vi "Stufentabelle umkehren.vi"(8 "error in (no error)":errorcluster caption="Fehler (Eingang, kein Fehler)") -> (0 "error out":errorcluster caption="Fehler (Ausgang)")   [LabVIEW 2020, in "Linearisierung v2.lvlib"]
uses:
  Linearisierung v2.lvlib
  Aktion Lin Daten aufarbeiten.ctl
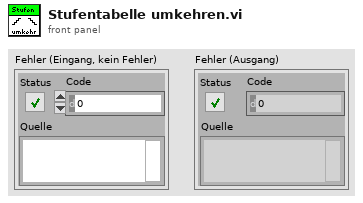
[diagram p1: front panel]
types:
  T1 = typedef "Linearisierung v2.lvlib/Aktion Lin Daten aufarbeiten.ctl" = enum16{"lesen", "Protkolldaten", "speichern", "laden", "EPA auswerten", "Tabelle schreiben", "Lin auswerten", "Tab init", "Stufentabelle", "EPA aktiviert", "Nachbehandlung laden", "Tabelle löschen", "Istwerte löschen", "Zeile löschen", "Zeile einfügen", "LIN aktiviert", "LIN/EPA aktiv laden", "EGAK Tab", "LIN übernehmen", "Tab init ohne Stufen"}
  T2 = typedef "Linearisierung v2.lvlib/Gasteiler.lvlib/Stufen Tabelle.ctl" = string[][]
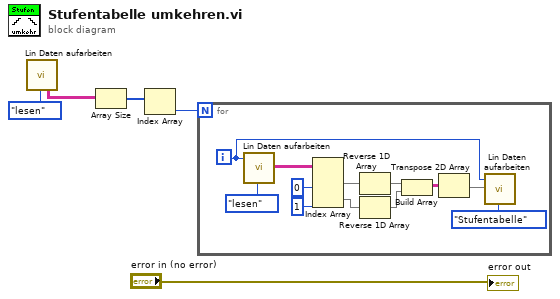
[diagram p0: block diagram]
diagram:
  n1 = call "Lin Daten aufarbeiten.vi"("Aktionen"=Aktion_Lin_Daten_aufarbeiten."lesen") -> ("TabellenArray"=w4:string[][][])  [unwired: 16 in, 10 out]
  n2 = Array Size(array=w4) -> (size(s)=w3:i32[])
  n3 = Index Array(array=w3) -> (element=w2:i32)  [unwired: 1 in]
  n4 = for {
    N: w2 -> [_]
    i -> [w15]
    n5 = call "Lin Daten aufarbeiten.vi"("Index (Seite)"=w15, "Aktionen"=Aktion_Lin_Daten_aufarbeiten."lesen") -> ("Stufen Tabelle"=w14:T2)  [unwired: 15 in, 10 out]
    n6 = Index Array(array=w14, index (col) #1=0 ("Deaktivierter Index (Spalte)"), index (col) #2=1 ("Index (Spalte)")) -> (element #1=w13:string[], element #2=w12:string[])  [unwired: 2 in]
    n7 = Reverse 1D Array(array=w13) -> (reversed array=w11:string[])
    n8 = Reverse 1D Array(array=w12) -> (reversed array=w10:string[])
    n9 = Build Array(w11, w10) -> (w9:string[][])
    n10 = Transpose 2D Array(2D array=w9) -> (transposed array=w6:string[][])
    n11 = call "Lin Daten aufarbeiten.vi"("Index (Seite)"=w15, "Stufen Tabelle"=w6, "Aktionen"=Aktion_Lin_Daten_aufarbeiten."Stufentabelle") -> ()  [unwired: 14 in, 11 out]
  }
  "error out" <- "error in (no error)"
